vi "Program Ramp.vi"(8 "error in (no error)":errorcluster, 9 "Ramp rate, K/min":dbl=1.0, 10 "Approach":T1, 11 "Mag Lab Temperature Controller in":refnum<class "Mag Lab Temperature Controller.lvclass">) -> (0 "error out":errorcluster, 3 "Mag Lab Temperature Controller out":refnum<class "Mag Lab Temperature Controller.lvclass">)   [LabVIEW 2015, in "Mag Lab Temperature Controller.lvclass"]
uses:
  Mag Lab Temperature Controller.lvclass
  Instruments/Neocera/Neocera Set Point Aproach.ctl
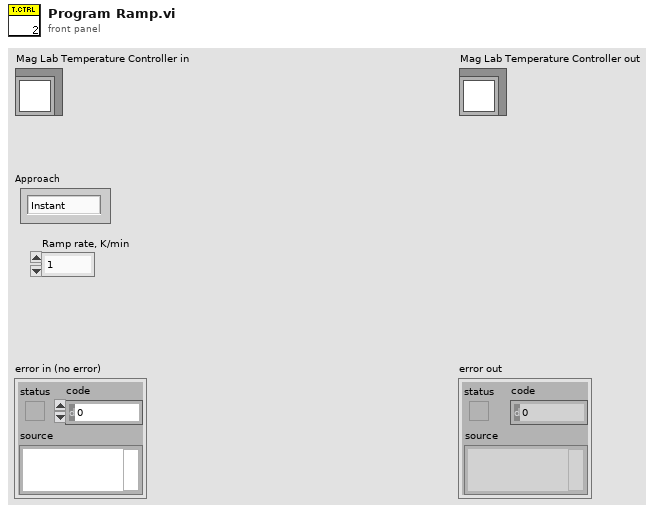
[diagram p1: front panel]
types:
  T1 = typedef "Neocera Set Point Aproach.ctl" = enum16{"Instant", "Ramp"}
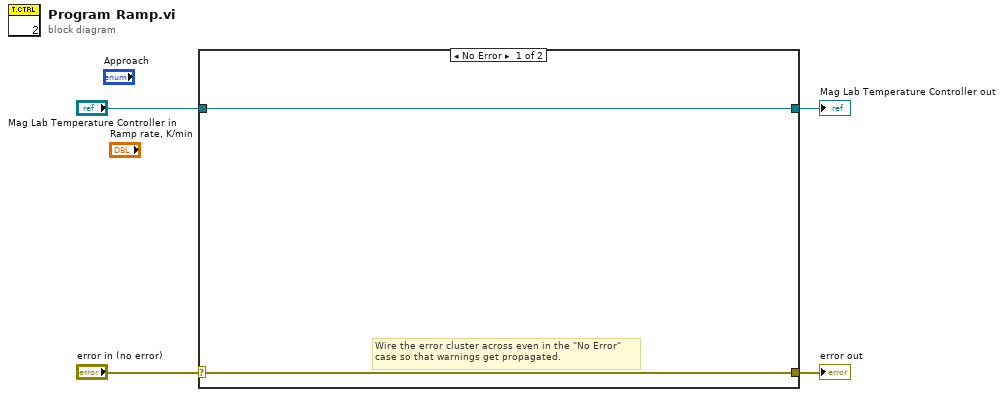
[diagram p0: block diagram]
diagram:
  n1 = case shown="No Error" "error in (no error)" {
    selector: "error in (no error)" -> [w5 w8]
    tunnel: [w5 w8] -> w3
    tunnel: [w6 w7] -> w1
    tunnel: "Mag Lab Temperature Controller in" -> [w6 w7]
    frame No Error {
      # "Wire the error cluster across even in the \"No Error\"\ncase so that warnings get propagated."
    }
    frame Error {
    }
  }
  "error out" <- w3
  "Mag Lab Temperature Controller out" <- w1
